vi "Autonomous_Execution.vi"(8 "error in":errorcluster, 10 "Autonomous_Queue":refnum<queue>, 11 "Queue Key":refnum<queue>) -> (2 "Done":bool)   [LabVIEW 2019]
uses:
  Queue_Key_Data.ctl
  RobotSubsystemsCluster.ctl
  Subsystems/Drive/Drive_Cluster.ctl
  Subsystems/Drive/Drive_States.ctl
  Subsystems/Intake/Intake_Cluster.ctl
  Subsystems/Intake/Intake_States.ctl
  Subsystems/Magazine/Magazine_Cluster.ctl
  Subsystems/Magazine/Magazine_States.ctl
  Subsystems/Flywheel/Flywheel_Cluster.ctl
  Subsystems/Flywheel/Flywheel_States.ctl
  Subsystems/Turret/Turret_Cluster.ctl
  Subsystems/Turret/Turret_States.ctl
  Globals/Magazine_Globals.vi
  Globals/Drive_Globals.vi
  Globals/Turret_Globals.vi
  Globals/Flywheel_Globals.vi
  Globals/Intake_Globals.vi
panel:
  in  "ignore previous (F)":bool
  in  "timeout in ms (-1)":i32=15
  out "notifiers out":refnum<notifier>[](array[refnum])
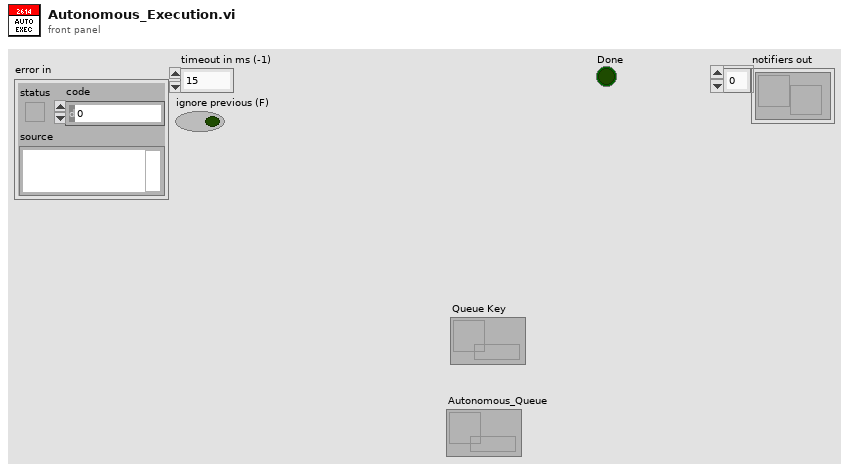
[diagram p1: front panel]
types:
  T1 = typedef "Queue_Key_Data.ctl" = cluster{"Operation Notifier":refnum<notifier>, "Subsystem":string, "Concurrent":bool}
  T2 = typedef "RobotSubsystemsCluster.ctl" = cluster{"Drive_Cluster":T3, "Intake_Cluster":T5, "Magazine_Cluster":T7, "Flywheel_Cluster":T9, "Turret_Cluster":T11}
  T3 = typedef "Drive_Cluster.ctl" = cluster{"Control_State":T4, "Angular_Throttle":dbl, "Linear_Throttle":dbl, "Torque_Changing":bool, "Step":dbl, "Parameter_1":dbl, "Parameter_2":dbl, "Parameter_3":dbl, "Parameter_4":dbl, "Auto_Notifier":refnum<notifier>}
  T4 = typedef "Drive_States.ctl" = enum16{"Percent_Voltage_Control", "Speed_Control", "Command_HeadingDistance", "Command_TurnToHeading"}
  T5 = typedef "Intake_Cluster.ctl" = cluster{"Control_State":T6, "Intake_On":bool, "Intake_Extended":bool, "Intake_Throttle":dbl, "Auto_Notifier":refnum<notifier>, "Parameter_1":dbl, "Parameter_2":dbl, "Step":dbl}
  T6 = typedef "Intake_States.ctl" = enum16{"Manual_Control", "Compliant_Intake", "Command_RunIntake"}
  T7 = typedef "Magazine_Cluster.ctl" = cluster{"Fire":bool, "Magazine_Throttle":dbl, "Control_States":T8, "Intake_Throttle":dbl, "Auto_Notifier":refnum<notifier>, "Parameter_1":dbl, "Parameter_2":dbl, "Step":dbl}
  T8 = typedef "Magazine_States.ctl" = enum16{"No-Op", "Loading", "Fire", "Unjam", "Manual_Percent_Voltage", "Manual_Speed_Control", "Command_Fire"}
  T9 = typedef "Flywheel_Cluster.ctl" = cluster{"Flywheel_Throttle":dbl, "Control_States":T10, "Auto_Speed":bool, "Flywheel_On":bool, "Parameter_1":dbl, "Parameter_2":dbl, "Auto_Notifier":refnum<notifier>, "Step":dbl}
  T10 = typedef "Flywheel_States.ctl" = enum16{"No-Op", "Percent_Voltage", "Speed_Control_Manual", "Speed_Control_Auto", "Command_SpinUp", "Command_SpinUpAuto"}
  T11 = typedef "Turret_Cluster.ctl" = cluster{"Auto-Target?":bool, "Control_State":T12, "Turret_Spin_Speed":dbl, "Turret_Spin_Speed_Control?":bool, "Step":dbl, "Parameter_1":dbl, "Parameter_2":dbl, "Parameter_3":dbl, "Auto_Notifier":refnum<notifier>}
  T12 = typedef "Turret_States.ctl" = enum16{"Manual_Percent_Voltage", "Manual_Speed_Control", "Auto-Target", "Command_TurnToPosition", "Command_Auto_Target"}
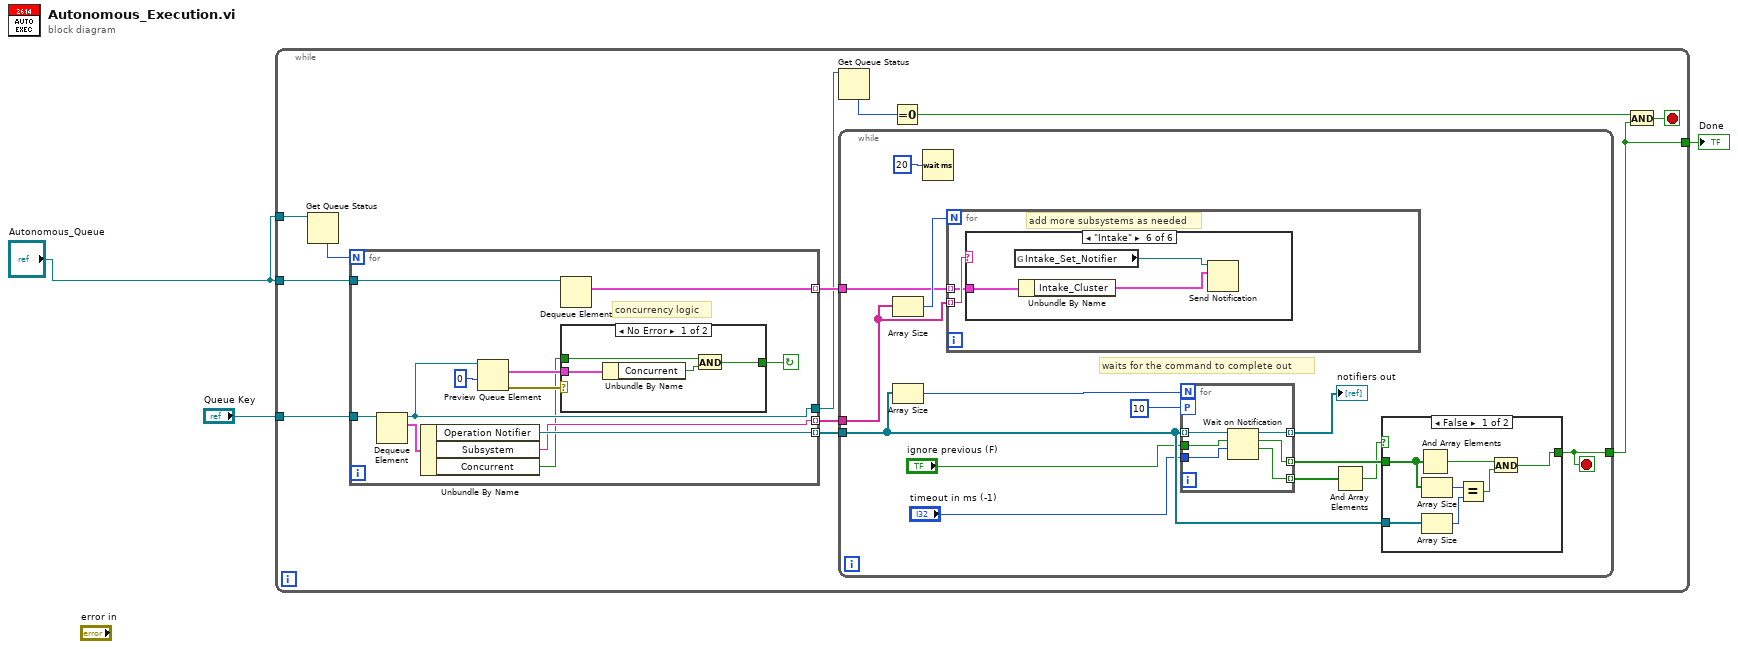
[diagram p0: block diagram]
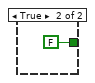
[diagram p2: hidden frame]
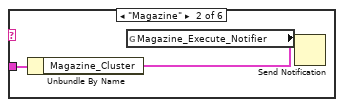
[diagram p4: hidden frame]
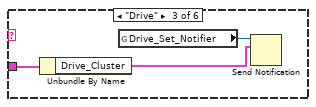
[diagram p5: hidden frame]
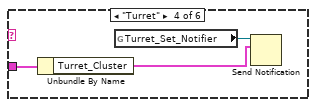
[diagram p6: hidden frame]
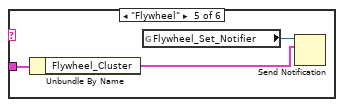
[diagram p7: hidden frame]
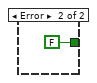
[diagram p8: hidden frame]
diagram:
  n1 = while {
    tunnel: "Queue Key" -> [w14]
    tunnel: "Autonomous_Queue" -> [w15]
    tunnel: "Autonomous_Queue" -> [w6]
    tunnel: [w4] -> w2
    stop <- w7 stop-if-true
    n2 = Get Queue Status(queue=w6) -> (# elements in queue=w9:i32)  [unwired: 2 in, 7 out]
    n3 = for {
      N: w9 -> [_]
      tunnel: w15 -> [w66]
      tunnel: w14 -> [w72]
      tunnel: [w63] -> w10 mode=indexing
      tunnel: [w67] -> w5
      tunnel: [w62] -> w12 mode=indexing
      tunnel: [w65] -> w11 mode=indexing
      stop <- w68 continue-if-true
      # "concurrency logic"
      n4 = Dequeue Element(queue=w72) -> (queue out=w67:refnum<queue>, element=w64:T1)  [unwired: 2 in, 2 out]
      n5 = Unbundle By Name(w64) -> ("Operation Notifier"=w63:refnum<notifier>, "Subsystem"=w62:string, "Concurrent"=w61:bool)
      n6 = Preview Queue Element(queue=w67, timeout in ms (-1)=0) -> (element=w71:T1, error out=w69:errorcluster)  [unwired: 1 in, 2 out]
      n7 = Dequeue Element(queue=w66) -> (element=w65:T2)  [unwired: 2 in, 3 out]
      n8 = case shown="No Error" w69 {
        tunnel: w71 -> [w74 _]
        tunnel: [w76 FALSE] -> w68
        tunnel: w61 -> [w75 _]
        frame No Error {
          n9 = Unbundle By Name(w74) -> ("Concurrent"=w73:bool)
          n10 = And(x=w75, y=w73) -> (x .and. y?=w76:bool)
        }
        frame Error {
        }
      }
    }
    n11 = Get Queue Status(queue=w5) -> (# elements in queue=w13:i32)  [unwired: 2 in, 7 out]
    n12 = while {
      tunnel: w12 -> [w24]
      tunnel: w11 -> [w23]
      tunnel: w10 -> [w25]
      tunnel: [w26] -> w4
      stop <- w26 stop-if-true
      # "waits for the command to complete out"
      n13 = Array Size(array=w24) -> (size(s)=w27:i32)
      n14 = Array Size(array=w25) -> (size(s)=w19:i32)
      n15 = Wait (ms)(milliseconds to wait=u32 20) -> ()  [unwired: 1 out]
      n16 = for {
        N: w27 -> [_]
        tunnel: w24 -> [w45] mode=indexing
        tunnel: w23 -> [w44] mode=indexing
        # "add more subsystems as needed"
        n17 = case shown="\"Intake\"" w45 {
          tunnel: w44 -> [_ w48 w51 w54 w56 w60]
          frame "No_Op", Default {
          }
          frame "Magazine" {
            n18 = Unbundle By Name(w48) -> ("Magazine_Cluster"=w47:T7)
            n19 = global read "Magazine_Globals.vi" "Magazine_Execute_Notifier"() -> (w46:refnum<notifier>)
            n20 = Send Notification(notification=w47, notifier=w46) -> ()  [unwired: 1 in, 2 out]
          }
          frame "Drive" {
            n21 = Unbundle By Name(w51) -> ("Drive_Cluster"=w50:T3)
            n22 = global read "Drive_Globals.vi" "Drive_Set_Notifier"() -> (w49:refnum<notifier>)
            n23 = Send Notification(notification=w50, notifier=w49) -> ()  [unwired: 1 in, 2 out]
          }
          frame "Turret" {
            n24 = Unbundle By Name(w54) -> ("Turret_Cluster"=w52:T11)
            n25 = global read "Turret_Globals.vi" "Turret_Set_Notifier"() -> (w53:refnum<notifier>)
            n26 = Send Notification(notification=w52, notifier=w53) -> ()  [unwired: 1 in, 2 out]
          }
          frame "Flywheel" {
            n27 = Unbundle By Name(w56) -> ("Flywheel_Cluster"=w55:T9)
            n28 = global read "Flywheel_Globals.vi" "Flywheel_Set_Notifier"() -> (w57:refnum<notifier>)
            n29 = Send Notification(notification=w55, notifier=w57) -> ()  [unwired: 1 in, 2 out]
          }
          frame "Intake" {
            n30 = global read "Intake_Globals.vi" "Intake_Set_Notifier"() -> (w58:refnum<notifier>)
            n31 = Unbundle By Name(w60) -> ("Intake_Cluster"=w59:T5)
            n32 = Send Notification(notification=w59, notifier=w58) -> ()  [unwired: 1 in, 2 out]
          }
        }
      }
      n33 = for {
        N: w19 -> [_]
        tunnel: w25 -> [w35] mode=indexing
        workers-P: 10 -> [_]
        tunnel: "timeout in ms (-1)" -> [w34]
        tunnel: "ignore previous (F)" -> [w33]
        tunnel: [w32] -> w22 mode=indexing
        tunnel: [w31] -> w29 mode=indexing
        tunnel: [w30] -> w17 mode=indexing
        n34 = Wait on Notification(notifier=w35, ignore previous (F)=w33, timeout in ms (-1)=w34) -> (notifier out=w32:refnum<notifier>, notification=w31:bool, timed out?=w30:bool)  [unwired: 1 in, 1 out]
      }
      "notifiers out" <- w22
      n35 = And Array Elements(Boolean array=w17) -> (logical AND=w28:bool)
      n36 = case shown="False" w28 {
        tunnel: [w41 FALSE] -> w26
        tunnel: w29 -> [w40 _]
        tunnel: w25 -> [w39 _]
        frame False {
          n37 = And Array Elements(Boolean array=w40) -> (logical AND=w42:bool)
          n38 = Array Size(array=w40) -> (size(s)=w38:i32)
          n39 = Array Size(array=w39) -> (size(s)=w37:i32)
          n40 = Equal?(x=w38, y=w37) -> (x = y?=w36:bool)
          n41 = And(x=w42, y=w36) -> (x .and. y?=w41:bool)
        }
        frame True {
        }
      }
    }
    n42 = Equal To 0?(x=w13) -> (x = 0?=w8:bool)
    n43 = And(x=w8, y=w4) -> (x .and. y?=w7:bool)
  }
  "Done" <- w2
